vi "VI Tree.vi"   [LabVIEW 2019, in "NI_Advanced HTTP Client.lvlib"]
uses:
  NI_Advanced HTTP Client.lvlib
  Session.lvclass
  Generic Request (Buffer).vi
  POST (Buffer).vi
  PATCH (Buffer).vi
  PUT (Buffer).vi
panel:
  # "See block diagram to browse the organization of the NI Advanced HTTP Client VIs."
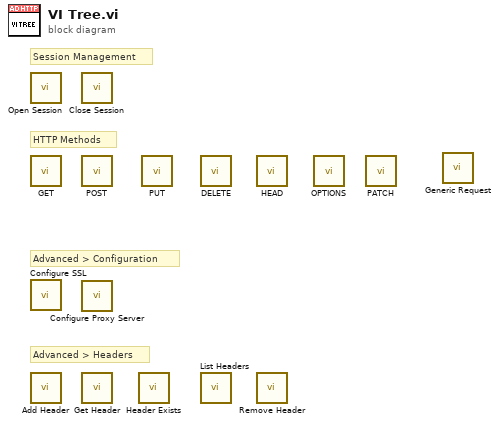
[diagram p0: block diagram]
diagram:
  # "Advanced > Headers"
  # "Advanced > Configuration"
  # "HTTP Methods"
  # "Session Management"
  n1 = call "Open Session.vi"() -> ()  [unwired: 10 in, 2 out]
  n2 = call "GET.vi"() -> ()  [unwired: 7 in, 5 out]
  n3 = call "Configure SSL.vi"() -> ()  [unwired: 10 in, 2 out]
  n4 = call "Add Header.vi"() -> ()  [unwired: 10 in, 2 out]
  n5 = call "Close Session.vi"() -> ()  [unwired: 11 in, 1 out]
  n6 = call-poly "POST.vi"() -> ()  [unwired: 7 in, 5 out]
  n7 = call "Configure Proxy Server.vi"() -> ()  [unwired: 10 in, 2 out]
  n8 = call "Get Header.vi"() -> ()  [unwired: 9 in, 3 out]
  n9 = call "Header Exists.vi"() -> ()  [unwired: 8 in, 4 out]
  n10 = call-poly "PUT.vi"() -> ()  [unwired: 7 in, 5 out]
  n11 = call "DELETE.vi"() -> ()  [unwired: 7 in, 5 out]
  n12 = call "List Headers.vi"() -> ()  [unwired: 9 in, 3 out]
  n13 = call "HEAD.vi"() -> ()  [unwired: 8 in, 4 out]
  n14 = call "Remove Header.vi"() -> ()  [unwired: 10 in, 2 out]
  n15 = call "OPTIONS.vi"() -> ()  [unwired: 7 in, 5 out]
  n16 = call-poly "PATCH.vi"() -> ()  [unwired: 7 in, 5 out]
  n17 = call-poly "Generic Request.vi"() -> ()  [unwired: 7 in, 5 out]
